vi "main elapsed time botó on off.vi"() -> ()   [LabVIEW 2019]
uses:
  Controls/Estats.ctl
panel:
  in  "OK Button":bool
  in  "Stop Button":bool
  out "Numeric":i32
  in  "stop":bool
  out "Boolean":bool
  # "fixar-se en la velocitat d'execució ara"
  # "botons per forçar el canvi d'estat"
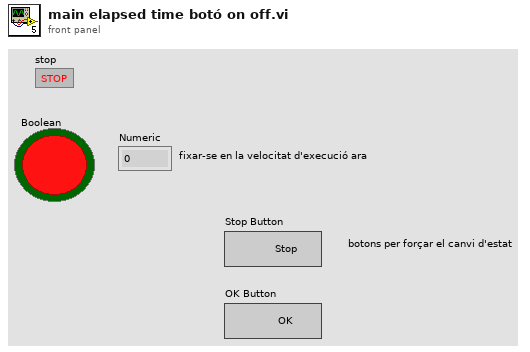
[diagram p1: front panel]
types:
  T1 = typedef "Estats.ctl" = enum16{"inicialitza", "Estat1", "Estat2"}
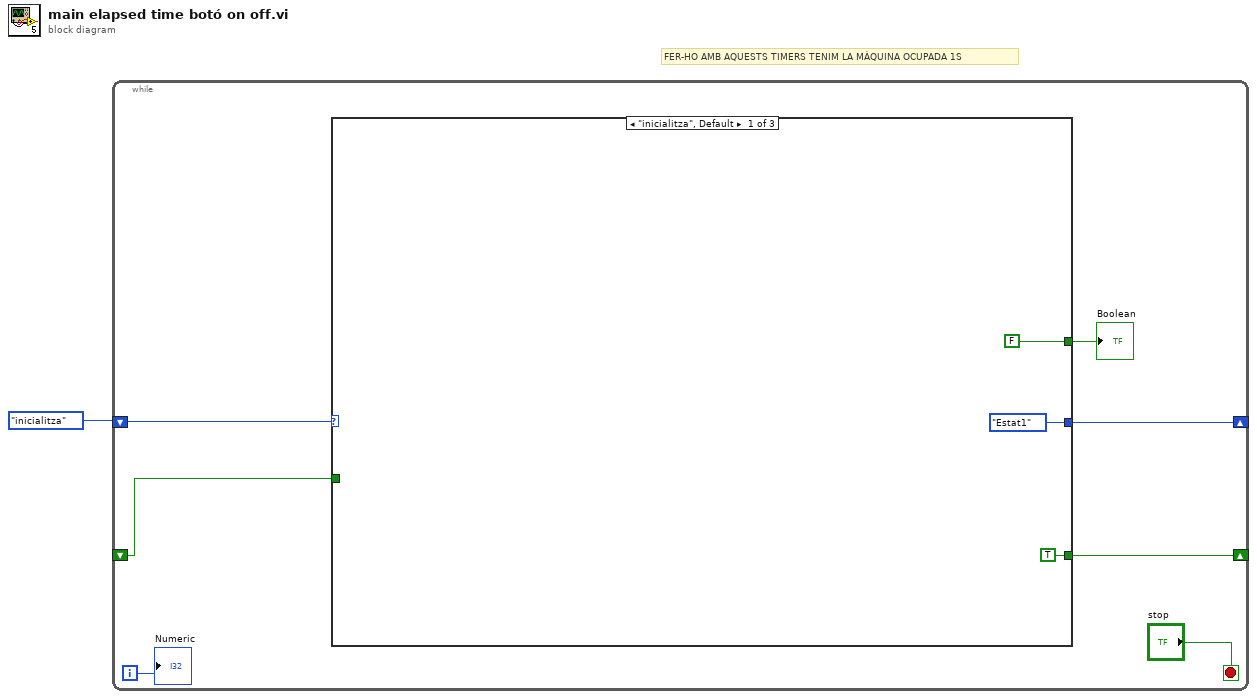
[diagram p0: block diagram]
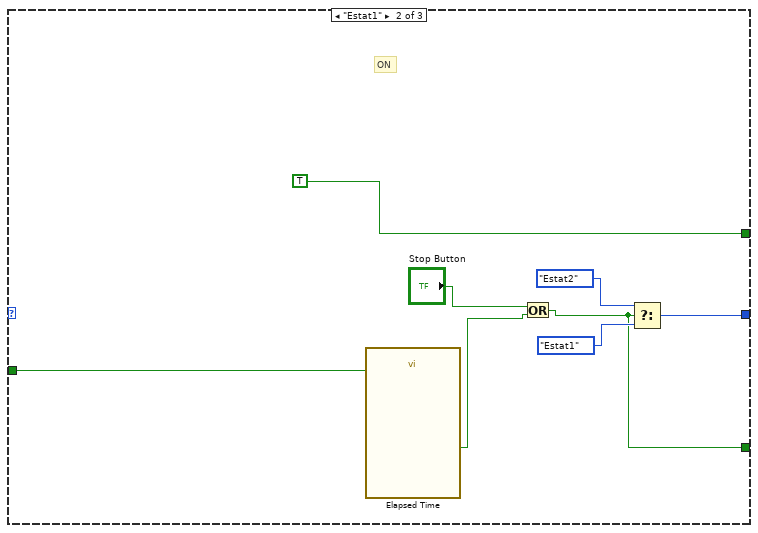
[diagram p2: hidden frame]
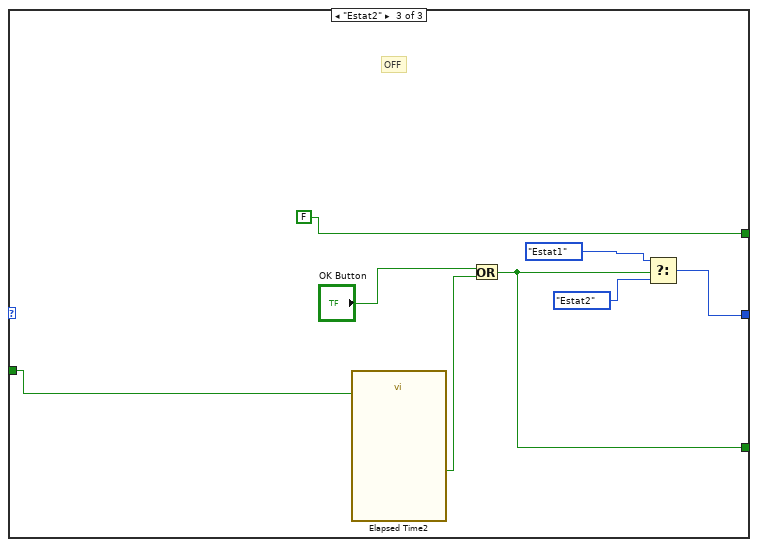
[diagram p3: hidden frame]
diagram:
  # "FER-HO AMB AQUESTS TIMERS TENIM LA MÀQUINA OCUPADA 1S"
  n1 = while {
    shift-right: [w7] -> _
    shift-left: Estats."inicialitza" ("Enum") -> [w8]
    shift-right: [w4] -> _
    shift-left: _ -> [w3]
    i -> [w2]
    stop <- "stop" stop-if-true
    n2 = case shown="\"inicialitza\", Default" w8 {
      tunnel: [Estats."Estat1" ("Enum") w16 w26] -> w7
      tunnel: [FALSE ("Boolean") TRUE ("Boolean") FALSE ("Boolean")] -> w5
      tunnel: [TRUE ("Time has Elapsed") w12 w20] -> w4
      tunnel: w3 -> [_ w15 w24]
      frame "inicialitza", Default {
      }
      frame "Estat1" {
        # "ON"
        n3 = call "Elapsed Time"("Reset"=w15) -> ("Time has Elapsed"=w14:bool)  [unwired: 11 in, 7 out]
        n4 = Or(x="Stop Button", y=w14) -> (x .or. y?=w12:bool)
        n5 = Select(t=Estats."Estat2" ("Enum"), s=w12, f=Estats."Estat1" ("Enum")) -> (s? t:f=w16:T1)
      }
      frame "Estat2" {
        # "OFF"
        n6 = call "Elapsed Time2"("Reset"=w24) -> ("Time has Elapsed"=w22:bool)  [unwired: 11 in, 7 out]
        n7 = Or(x="OK Button", y=w22) -> (x .or. y?=w20:bool)
        n8 = Select(t=Estats."Estat1" ("Enum"), s=w20, f=Estats."Estat2" ("Enum")) -> (s? t:f=w26:T1)
      }
    }
    "Boolean" <- w5
    "Numeric" <- w2
  }
